vi "Write WebSocket.vi"(8 "error in (no error)":errorcluster, 10 "Socket":refnum<class "Socket.lvclass">, 11 "Connection Handler in":refnum<class "Connection Handler.lvclass">) -> (0 "error out":errorcluster, 3 "Connection Handler out":refnum<class "Connection Handler.lvclass">)   [LabVIEW 2017, in "Connection Handler.lvlib" / "Connection Handler.lvclass"]
uses:
  Connection Handler.lvclass
  <vilib>/MediaMongrels Ltd/WebSockets/Sockets/Socket/Socket.lvclass
  Connection Handler.lvclass/Connection Handler.ctl
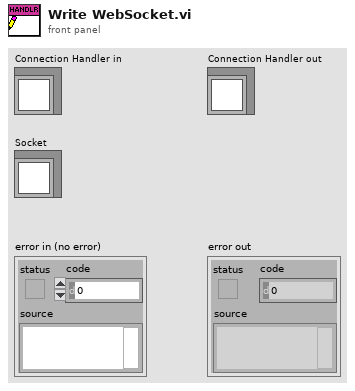
[diagram p1: front panel]
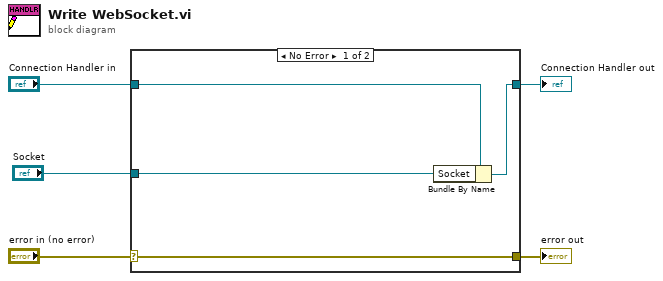
[diagram p0: block diagram]
diagram:
  n1 = case shown="No Error" "error in (no error)" {
    selector: "error in (no error)" -> [w9 w10]
    tunnel: [w9 w10] -> w4
    tunnel: [w7 w11] -> w2
    tunnel: "Connection Handler in" -> [w8 w11]
    tunnel: "Socket" -> [w6 _]
    frame No Error {
      n2 = Bundle By Name(cluster=w8, "Socket"=w6) -> (w7:refnum<class "Connection Handler.lvclass">)
    }
    frame Error {
    }
  }
  "error out" <- w4
  "Connection Handler out" <- w2
